vi "RM.getReservationList.vi"(5 "Resource Type":T1, 7 "Direction":T2, 8 "error in":errorcluster, 11 "reservation DB in":variant) -> (0 "error out":errorcluster, 1 "reservers":string[](array[string]), 2 "names in bitfile":string[](array[string]), 3 "reservation DB out":variant)   [LabVIEW 2016, in "FPGA Addon Shared.lvlib"]
uses:
  FPGA Addon Shared.lvlib
  RM.resourceDirection.ctl
  RM.resourceType.ctl
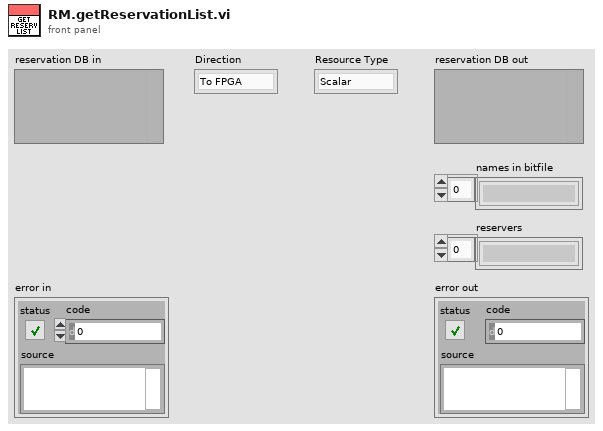
[diagram p1: front panel]
types:
  T1 = typedef "FPGA Addon Shared.lvlib/RM.resourceType.ctl" = enum16{"Scalar", "Waveform"}
  T2 = typedef "FPGA Addon Shared.lvlib/RM.resourceDirection.ctl" = enum16{"To FPGA", "From FPGA"}
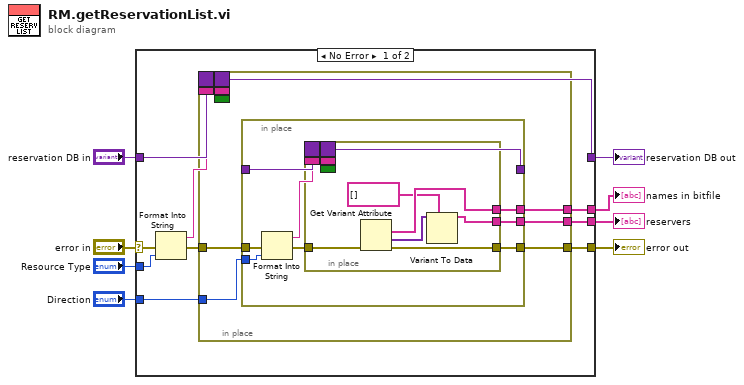
[diagram p0: block diagram]
diagram:
  n1 = case shown="No Error" "error in" {
    selector: "error in" -> [w12 w43]
    tunnel: "reservation DB in" -> [w18 w44]
    tunnel: "Direction" -> [w17 _]
    tunnel: [w16 w44] -> w3
    tunnel: "Resource Type" -> [w15 _]
    tunnel: [w11 w43] -> w4
    tunnel: [w10 _] -> w2
    tunnel: [w9 _] -> w1
    frame No Error {
      n2 = Format Into String(error in=w12, w15) -> (resulting string=w14:string, error out=w13:errorcluster)  [unwired: 2 in]
      n3 = in-place {
        in-place-border: w17 -> [w25]
        in-place-border: w13 -> [w22]
        in-place-border: [w21] -> w11
        in-place-border: [w20] -> w10
        border: w18 -> [_]
        border: w14 -> [_]
        border: [_] -> w16
        border: _ -> [_]
        border: _ -> [_]
        in-place-border: [w19] -> w9
        n4 = in-place {
          in-place-border: w25 -> [w32]
          in-place-border: w24 -> [w34]
          in-place-border: [w33] -> w23
          in-place-border: w22 -> [w30]
          in-place-border: [w28] -> w21
          in-place-border: [w27] -> w20
          in-place-border: [w26] -> w19
          n5 = Format Into String(error in=w30, w32) -> (resulting string=w31:string, error out=w29:errorcluster)  [unwired: 2 in]
          n6 = in-place {
            in-place-border: w29 -> [w41]
            in-place-border: [w40] -> w28
            in-place-border: [w39] -> w27
            border: w34 -> [_]
            border: w31 -> [_]
            border: [_] -> w33
            border: _ -> [_]
            border: _ -> [_]
            in-place-border: [w35] -> w26
            n7 = Get Variant Attribute(Variant=w38, error in=w41) -> (duplicate Variant=w42:variant, names=w39:string[], values=w37:variant[], error out=w40:errorcluster)  [unwired: 2 in]
            n8 = Variant To Data(type=string[] [] ("name"), Variant=w37) -> (data=w35:string[])  [unwired: 1 in, 1 out]
          }
        }
      }
    }
    frame Error {
    }
  }
  "reservation DB out" <- w3
  "error out" <- w4
  "names in bitfile" <- w2
  "reservers" <- w1
